vi "Remove Channel.vi"(7 "BLRL Type":T1, 8 "error in (no error)":errorcluster, 10 "Channel":string, 11 "BluelinesRedlines in":refnum<class "BluelinesRedlines.lvclass">) -> (0 "error out":errorcluster, 3 "BluelinesRedlines out":refnum<class "BluelinesRedlines.lvclass">)   [LabVIEW 2020, in "VolatusGUIElements.lvlib" / "BluelinesRedlines.lvclass"]
uses:
  BluelinesRedlines.lvclass
  VolatusGUI/BluelinesRedlines Source/BLRL Type.ctl
  BluelinesRedlines.lvclass/BluelinesRedlines.ctl
  User BluelinesRedlines/User BluelinesRedlines.lvclass
  C:/dev/lv20CE/relink/lv-volatus/VolatusGUI/BluelinesRedlines Source/BluelinesRedlines Source.lvclass
  VolatusGUI/BluelinesRedlines Source/BluelinesRedlines Source.lvclass
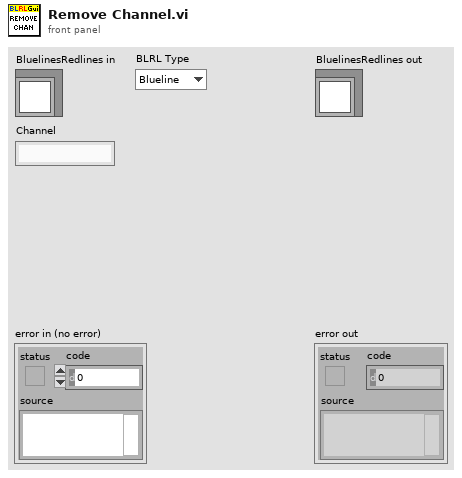
[diagram p1: front panel]
types:
  T1 = typedef "VolatusGUI.lvlib/BluelinesRedlines Source.lvclass/BLRL Type.ctl" = enum16{"Blueline", "Redline"}
  T2 = map{string, refnum<class "BluelinesRedlines Source.lvclass">}
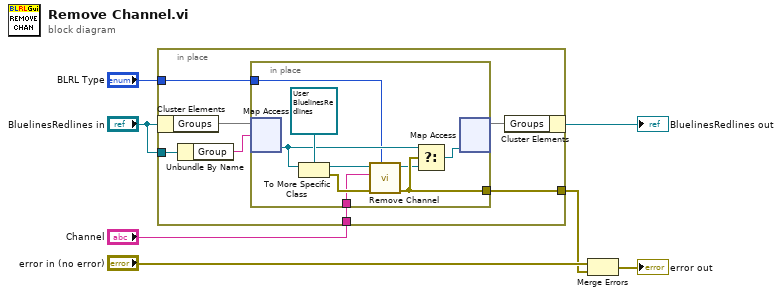
[diagram p0: block diagram]
diagram:
  n1 = in-place {
    in-place-border: "BluelinesRedlines in" -> [w14]
    in-place-border: "Channel" -> [w10]
    in-place-border: "BLRL Type" -> [w9]
    in-place-border: [w8] -> w1
    n2 = in-place-cluster #1("BluelinesRedlines in") -> ("Groups"=w13:T2)
    n3 = Unbundle By Name(w14) -> ("Group"=w12:string)
    n4 = in-place {
      in-place-border: w10 -> [w17]
      in-place-border: w9 -> [w16]
      in-place-border: [w23] -> w8
      n5 = in-place-map #2(w13, w12) -> (w20:refnum<class "BluelinesRedlines Source.lvclass">)  [unwired: 1 in, 1 out]
      n6 = To More Specific Class(target class=refnum<class "User BluelinesRedlines.lvclass"> refnum ("VolatusGUIElements.lvlib:User BluelinesRedlines.lvclass"), reference=w20) -> (specific class reference=w18:refnum<class "User BluelinesRedlines.lvclass">, error out=w22:errorcluster)  [unwired: 1 in]
      n7 = call "Remove Channel.vi"("Type"=w16, "error in (no error)"=w22, "Channel Name"=w17, "User BluelinesRedlines in"=w18) -> ("error out"=w23:errorcluster, "User BluelinesRedlines out"=w15:refnum<class "User BluelinesRedlines.lvclass">)  [unwired: 6 in]
      n8 = Select(t=w20, s=w23, f=w15) -> (s? t:f=w19:refnum<class "BluelinesRedlines Source.lvclass">)
      n9 = in-place-map #2(w19) -> (w11:T2)  [unwired: 1 in, 2 out]
    }
    n10 = in-place-cluster #1("Groups"=w11) -> (→"BluelinesRedlines out":refnum<class "BluelinesRedlines.lvclass">)
  }
  n11 = Merge Errors("error in (no error)", w1) -> (→"error out":errorcluster)
